vi "多曲线chart显示.vi"() -> ()   [LabVIEW 2014]
doc: "该范例演示了在不同的图表中绘制不同类型的数据。图表可一次输入一个点，也可一次输入多个点。图表也可分格显示曲线或层叠显示曲线。右键单击图表，选择“高级>>刷新模式”，可更改刷新模式（带状图表、示波器图表和扫描图）。"
panel:
  in  "选项卡控件":enum32{"簇（多条曲线）", "簇数组（多条曲线）", "二维数组（多条曲线）"}(tab)
  out "簇（多条曲线）":cluster{dbl, dbl}(graph)
  out "簇数组（多条曲线）":cluster{dbl, dbl}[](graph)
  out "二维数组（多条曲线）":dbl[][](graph)
  in  "停止":bool
  # "概述：演示波形图表的数据类型和刷新模式。\n操作步骤：\n1. 运行VI。\n2. 切换不同的选项卡查看不同波形图表的外观。\n3. 单击停止停止VI。"
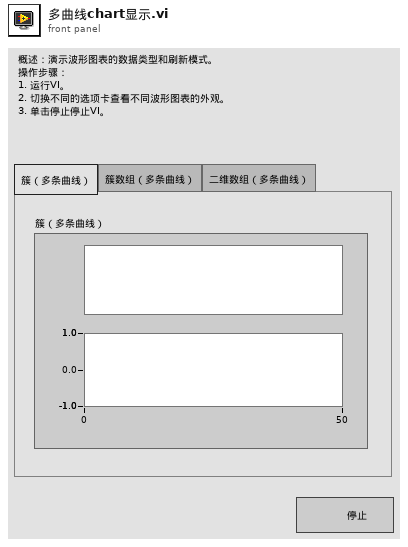
[diagram p1: front panel]
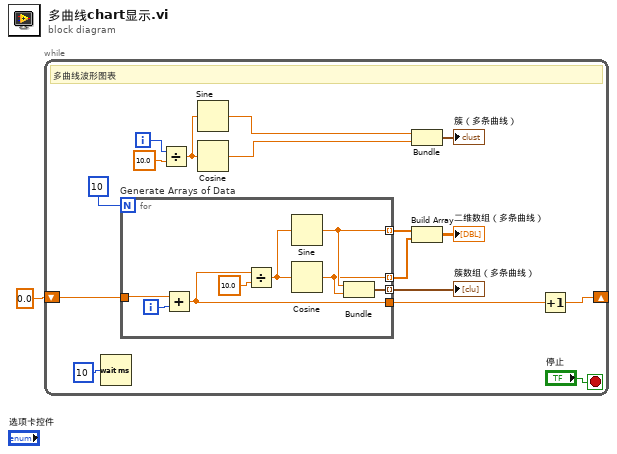
[diagram p0: block diagram]
diagram:
  n1 = while {
    shift-right: [w4] -> _
    shift-left: 0.0 -> [w6]
    i -> [w17]
    stop <- "停止" stop-if-true
    # "多曲线波形图表"
    n2 = Wait (ms)(milliseconds to wait=u32 10 ("millisecond multiple")) -> ()  [unwired: 1 out]
    n3 = for "Generate Arrays of Data" {
      N: 10 ("# of Pts/update") -> [_]
      tunnel: [w24] -> w3 mode=indexing
      tunnel: [w23] -> w9 mode=indexing
      tunnel: [w20] -> w2 mode=indexing
      tunnel: w6 -> [w19]
      tunnel: [w18] -> w5
      i -> [w22]
      n4 = Add(x=w19, y=w22) -> (x+y=w18:dbl)
      n5 = Divide(x=w18, y=10.0) -> (x/y=w25:dbl)
      n6 = Sine(x=w25) -> (sin(x)=w24:dbl)
      n7 = Cosine(x=w25) -> (cos(x)=w20:dbl)
      n8 = Bundle(w24, w20) -> (w23:cluster{dbl, dbl})  [unwired: 1 in]
    }
    "簇数组（多条曲线）" <- w9
    n9 = Divide(x=w17, y=10.0) -> (x/y=w16:dbl)
    n10 = Sine(x=w16) -> (sin(x)=w15:dbl)
    n11 = Cosine(x=w16) -> (cos(x)=w14:dbl)
    n12 = Bundle(w15, w14) -> (→"簇（多条曲线）":cluster{dbl, dbl})  [unwired: 1 in]
    n13 = Build Array(w3, w2) -> (→"二维数组（多条曲线）":dbl[][])
    n14 = Increment(x=w5) -> (x+1=w4:dbl)
  }
